vi "Generate RPC Methods.vi"(7 "RPC Method Parameters":T1[](array[typedef]), 8 "error in (no error)":errorcluster, 11 "Server class in":refnum<vi>) -> (0 "error out":errorcluster, 3 "Server class out":refnum<vi>)   [LabVIEW 2019, in "gRPC Scripting Tools.lvlib"]
uses:
  gRPC Scripting Tools.lvlib
  TypeDefs/RPC Method Parameters.ctl
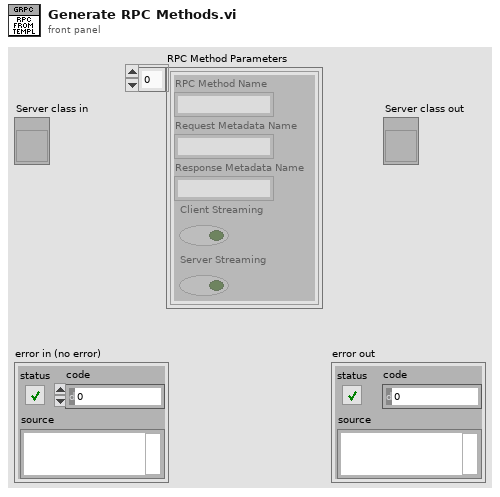
[diagram p1: front panel]
types:
  T1 = typedef "gRPC Scripting Tools.lvlib/RPC Method Parameters.ctl" = cluster{"RPC Method Name":string, "Request Metadata Name":string, "Response Metadata Name":string, "Client Streaming":bool, "Server Streaming":bool}
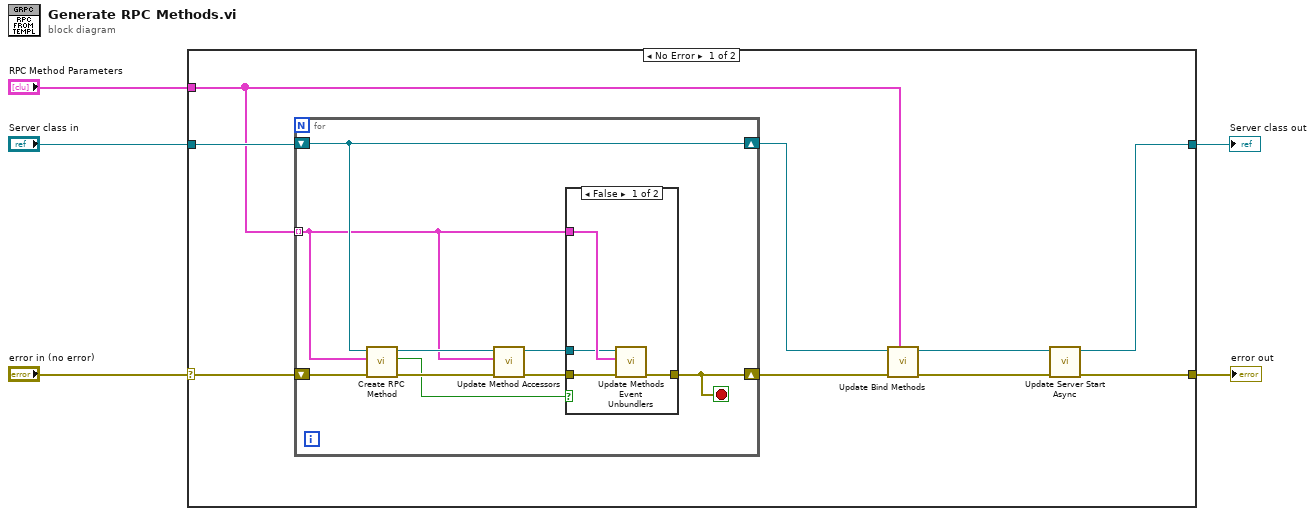
[diagram p0: block diagram]
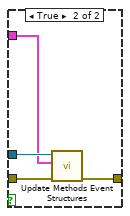
[diagram p2: hidden frame]
diagram:
  n1 = case shown="No Error" "error in (no error)" {
    selector: "error in (no error)" -> [w14 w33]
    tunnel: [w8 w33] -> w5
    tunnel: "Server class in" -> [w13 w32]
    tunnel: [w6 w32] -> w2
    tunnel: "RPC Method Parameters" -> [w11 _]
    frame No Error {
      n2 = for {
        tunnel: w11 -> [w16] mode=indexing
        shift-right: [w22] -> w12
        shift-left: w14 -> [w23]
        shift-right: [w21] -> w10
        shift-left: w13 -> [w21]
        stop <- w22 stop-if-true
        n3 = call "Create RPC Method.vi"("error in (no error)"=w23, "RPC Method Parameters"=w16, "Server class in"=w21) -> ("error out"=w18:errorcluster, "Newly created ?"=w15:bool, "Server class out"=w20:refnum<vi>)  [unwired: 6 in]
        n4 = call "Update Method Accessors.vi"("error in (no error)"=w18, "RPC Method Parameters"=w16, "Server class in"=w20) -> ("error out"=w17:errorcluster, "Server class out"=w19:refnum<vi>)  [unwired: 7 in]
        n5 = case shown="False" w15 {
          tunnel: w17 -> [w27 w31]
          tunnel: w19 -> [w24 w30]
          tunnel: w16 -> [w25 w29]
          tunnel: [w26 w28] -> w22
          frame False {
            n6 = call "Update Methods Event Unbundlers.vi"("error in (no error)"=w27, "RPC Method Parameters"=w25, "LVClassLibrary in"=w24) -> ("error out"=w26:errorcluster)  [unwired: 7 in, 1 out]
          }
          frame True {
            n7 = call "Update Methods Event Structures.vi"("error in (no error)"=w31, "RPC Method Parameters"=w29, "LVClassLibrary in"=w30) -> ("error out"=w28:errorcluster)  [unwired: 7 in, 1 out]
          }
        }
      }
      n8 = call "Update Bind Methods.vi"("RPC Method Parameters"=w11, "error in (no error)"=w12, "Server class in"=w10) -> ("error out"=w9:errorcluster, "Server class out"=w7:refnum<vi>)  [unwired: 7 in]
      n9 = call "Update Server Start Async.vi"("error in (no error)"=w9, "Server class in"=w7) -> ("error out"=w8:errorcluster, "Server class out"=w6:refnum<vi>)  [unwired: 8 in]
    }
    frame Error {
    }
  }
  "error out" <- w5
  "Server class out" <- w2
